vi "AVS_GetScopeData.vi"(0 "a_hDevice":i32, 7 "a_pTimeLabel":u32, 11 "a_pSpectrum":dbl[](array[numeric])) -> (4 "Output Value":i32, 8 "a_pTimeLabel":u32, 15 "a_pSpectrum":dbl[](array[numeric]))   [LabVIEW 2020]
uses:
  AvaSpecX64-DLL_9.4/avaspecx64.dll
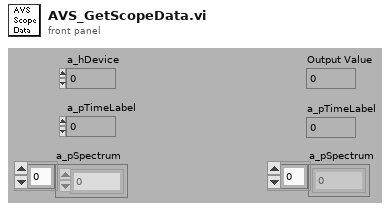
[diagram p1: front panel]
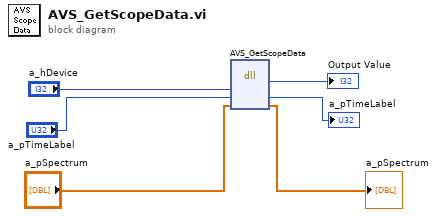
[diagram p0: block diagram]
diagram:
  n1 = dll-call lib="C:/AvaSpecX64-DLL_9.4/avaspecx64.dll" fn="AVS_GetScopeData"("a_hDevice"="a_hDevice", "a_pTimeLabel"="a_pTimeLabel", "a_pSpectrum"="a_pSpectrum") -> ("return type"=→"Output Value":i32, "a_pTimeLabel"=→"a_pTimeLabel":u32, "a_pSpectrum"=→"a_pSpectrum":dbl[])  [unwired: 4 in, 2 out]
